vi "Find Channel.vi"(8 "error in":errorcluster, 10 "hardwareChannel":i32, 11 "item ref in":T1 format="%.0x") -> (0 "error out":errorcluster, 2 "Found":bool, 3 "item ref out":T1 format="%.0x")   [LabVIEW 2020, in "Communication Bus Template Scripting.lvlib"]
uses:
  <vilib>/NI VeriStand/Custom Device API/Custom Device Item Ref.ctl
  Constants.vi
  <vilib>/NI VeriStand/Custom Device Tools/Custom Device Utility Library/NI VeriStand - Search for All Items by GUID.vi
  <vilib>/NI VeriStand/Custom Device API/Get Item Property (U16).vi
  Communication Bus Template Scripting.lvlib
  <vilib>/NI VeriStand/Custom Device API/Custom Device API.lvlib
  <vilib>/NI VeriStand/Custom Device Tools/Custom Device Utility Library/Custom Device Utility Library.lvlib
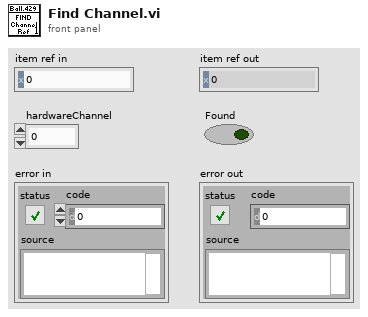
[diagram p1: front panel]
types:
  T1 = typedef "Custom Device API.lvlib/Custom Device Item Ref.ctl" = u64
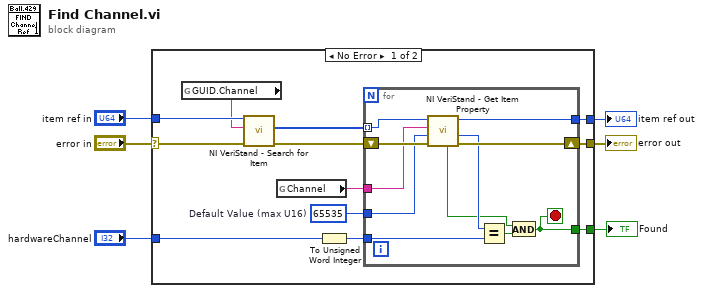
[diagram p0: block diagram]
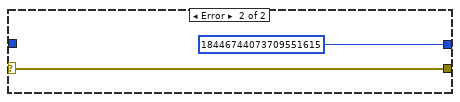
[diagram p2: hidden frame]
diagram:
  n1 = case shown="No Error" "error in" {
    selector: "error in" -> [w12 w31]
    tunnel: "hardwareChannel" -> [w18 _]
    tunnel: [w17 T1 18446744073709551615 ("Item Ref")] -> w5
    tunnel: [w16 w31] -> w4
    tunnel: "item ref in" -> [w15 _]
    tunnel: [w13 _] -> w2
    frame No Error {
      w9 = u16 65535  # Default Value (max U16)
      n2 = global read "Constants.vi" "GUID.Channel"() -> (w8:string)
      n3 = call-poly <vilib>:"NI VeriStand - Search for Item.vi"("error in"=w12, "Item GUID"=w8, "Section Ref in"=w15) -> ("error out"=w14:errorcluster, "Item Refs"=w10:T1[])  [unwired: 5 in, 2 out]
      n4 = global read "Constants.vi" "Channel"() -> (w7:string)
      n5 = To Unsigned Word Integer(number=w18) -> (unsigned 16bit integer=w11:u16)
      n6 = for {
        tunnel: w11 -> [w25]
        tunnel: [w29] -> w17
        shift-right: [w28] -> w16
        shift-left: w14 -> [w27]
        tunnel: w10 -> [w24] mode=indexing
        tunnel: [w21] -> w13
        tunnel: w9 -> [w20]
        tunnel: w7 -> [w19]
        stop <- w21 stop-if-true
        n7 = call-poly <vilib>:"NI VeriStand - Get Item Property.vi"("error in (no error)"=w27, "Default Value"=w20, "Property Name"=w19, "Item Ref in"=w24) -> ("error out"=w28:errorcluster, "Value"=w26:u16, "Item Ref out"=w29:T1, "Found?"=w22:bool)  [unwired: 4 in]
        n8 = Equal?(x=w26, y=w25) -> (x = y?=w23:bool)
        n9 = And(x=w22, y=w23) -> (x .and. y?=w21:bool)
      }
    }
    frame Error {
    }
  }
  "item ref out" <- w5
  "error out" <- w4
  "Found" <- w2
